vi "10_NOV_COMMAND_loop.vi"() -> ()   [LabVIEW 2020]
uses:
  <instrlib>/Agilent B2900 Series/Agilent B2900 Series.lvlib
panel:
  in  "VISA resource name":refnum<visa-resource-name>="USB0::0x0957::0x8E18::MY51140695::INSTR"
  out "Waveform Chart":dbl(graph)
  in  "stop":bool
  out "COMMAND":string
  in  "Measure":enum16{"Current", "Voltage", "Resistance"}(ring)
  in  "Source Voltage(V)":dbl
  in  "Channel":u16(ring) items=["", "1", "2"]
  out "Measurement":dbl
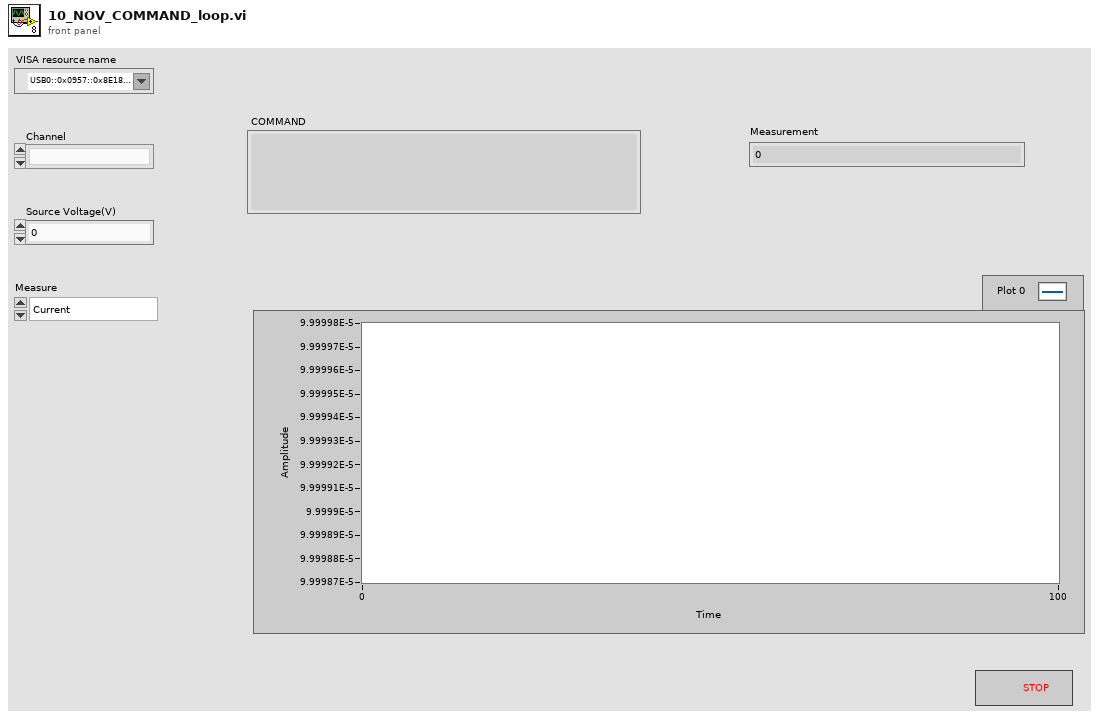
[diagram p1: front panel]
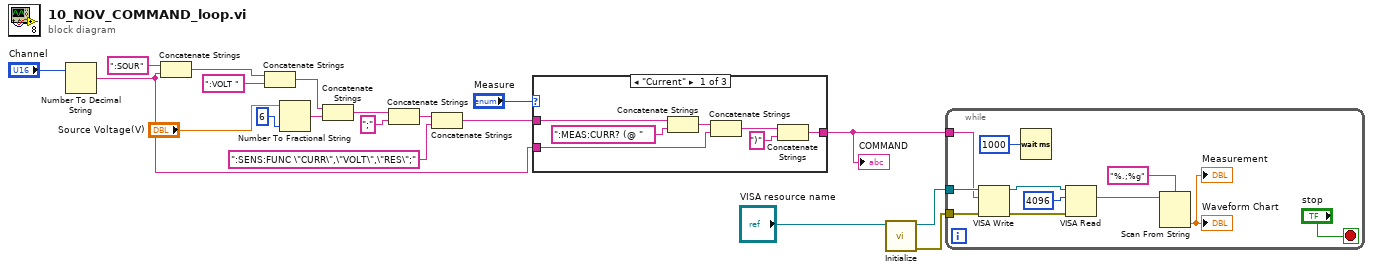
[diagram p0: block diagram]
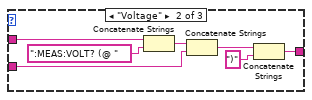
[diagram p2: hidden frame]
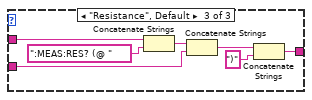
[diagram p3: hidden frame]
diagram:
  n1 = Number To Decimal String(number="Channel") -> (decimal integer string=w4:string)  [unwired: 1 in]
  n2 = Concatenate Strings(":SOUR", w4) -> (w16:string)
  n3 = Concatenate Strings(w16, ":VOLT ") -> (w14:string)
  n4 = Number To Fractional String(number="Source Voltage(V)", precision (6)=i16 6) -> (F-format string=w9:string)  [unwired: 2 in]
  n5 = Concatenate Strings(w14, w9) -> (w13:string)
  n6 = Concatenate Strings(w13, ";" ("string")) -> (w8:string)
  n7 = Concatenate Strings(w8, ":SENS:FUNC \"CURR\",\"VOLT\",\"RES\";") -> (w5:string)
  n8 = case shown="\"Current\"" "Measure" {
    tunnel: w5 -> [w22 w33 w36]
    tunnel: w4 -> [w21 w30 w35]
    tunnel: [w20 w27 w34] -> w3
    frame "Current" {
      n9 = Concatenate Strings(w22, ":MEAS:CURR? (@ " ("string")) -> (w25:string)
      n10 = Concatenate Strings(w25, w21) -> (w24:string)
      n11 = Concatenate Strings(w24, ")" ("string")) -> (w20:string)
    }
    frame "Voltage" {
      n12 = Concatenate Strings(w33, ":MEAS:VOLT? (@ " ("string")) -> (w31:string)
      n13 = Concatenate Strings(w31, w30) -> (w29:string)
      n14 = Concatenate Strings(w29, ")" ("string")) -> (w27:string)
    }
    frame "Resistance", Default {
      n15 = Concatenate Strings(w36, ":MEAS:RES? (@ " ("string")) -> (w39:string)
      n16 = Concatenate Strings(w39, w35) -> (w38:string)
      n17 = Concatenate Strings(w38, ")" ("string")) -> (w34:string)
    }
  }
  "COMMAND" <- w3
  n18 = call <instrlib>:"Initialize.vi"("VISA resource name"="VISA resource name") -> ("error out"=w2:errorcluster, "VISA resource name out"=w18:refnum<visa-resource-name>)  [unwired: 9 in]
  n19 = while {
    tunnel: w18 -> [w48]
    tunnel: w3 -> [w45]
    tunnel: w2 -> [w44]
    stop <- "stop" stop-if-true
    n20 = VISA Write(VISA resource name=w48, write buffer=w45, error in (no error)=w44) -> (VISA resource name out=w50:refnum<visa-resource-name>, error out=w49:errorcluster)  [unwired: 1 out]
    n21 = Wait (ms)(milliseconds to wait=u32 1000) -> ()  [unwired: 1 out]
    n22 = VISA Read(VISA resource name=w50, byte count=u32 4096, error in (no error)=w49) -> (read buffer=w46:string)  [unwired: 3 out]
    n23 = Scan From String(format string="%.;%g", input string=w46) -> (output 1=→"Measurement" →"Waveform Chart":dbl)  [unwired: 3 in, 3 out]
  }
